vi "deltaHRT.vi"(9 "data input":T3, 10 "Coagulant":T1={"flocculator volume (L)"=100.0, "clarifier volume (L)"=0.0, "dose updates per HRT"=0, "target clarified turbidity (NTU)"=0.3, "Coagulant mode"=enum."manual", "Coag dose [mg/L]"=0.0, "pump mL/rev"=0.0, "clarifier flow [L/s]"=0.5, "min Coag dose [mg/L]"=0.0, "max Coag dose [mg/L]"=0.0, "Steps"=3, "HRT response delay"=1, "Ku*"=1.0} {"HRT response delay" min=1 max=10 step=1; "Steps" min=3 step=1; "clarifier flow [L/s]" min=0.0001 max=1.0 step=0.0001; "target clarified turbidity (NTU)" min=0.1 max=5.0 step=0.01; "dose updates per HRT" min=1 max=100 step=1}, 11 "seconds since 1Jan1904":timestamp) -> (1 "new interval":bool, 2 "sum HRT since dose change":dbl, 3 "total HRT since startup":dbl)   [LabVIEW 2015]
uses:
  coag.ctl
  coag model data.ctl
  model type.ctl
panel:
  out "delta HRT":dbl
  # "min"
  # "max"
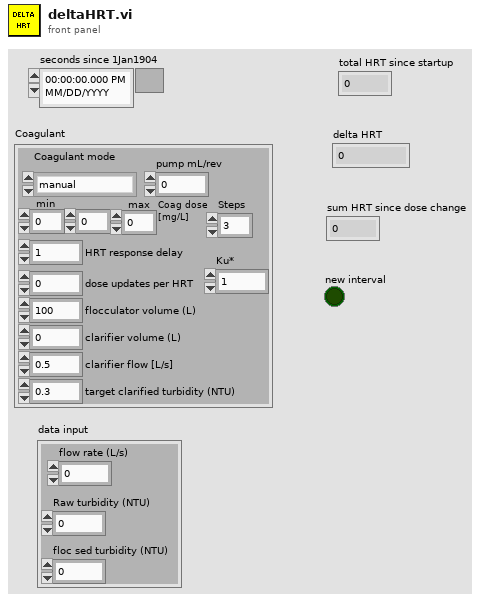
[diagram p1: front panel]
types:
  T1 = typedef "coag.ctl" = cluster{"flocculator volume (L)":dbl, "clarifier volume (L)":dbl, "dose updates per HRT":u16, "target clarified turbidity (NTU)":dbl, "Coagulant mode":T2, "Coag dose [mg/L]":dbl, "pump mL/rev":dbl, "clarifier flow [L/s]":dbl, "min Coag dose [mg/L]":dbl, "max Coag dose [mg/L]":dbl, "Steps":u16, "HRT response delay":u32, "Ku*":dbl}
  T2 = typedef "model type.ctl" = enum16{"manual", "ramp", "simple corrector", "linear regression"}
  T3 = typedef "coag model data.ctl" = cluster{"flow rate (L/s)":dbl, "Raw turbidity (NTU)":dbl, "floc sed turbidity (NTU)":dbl}
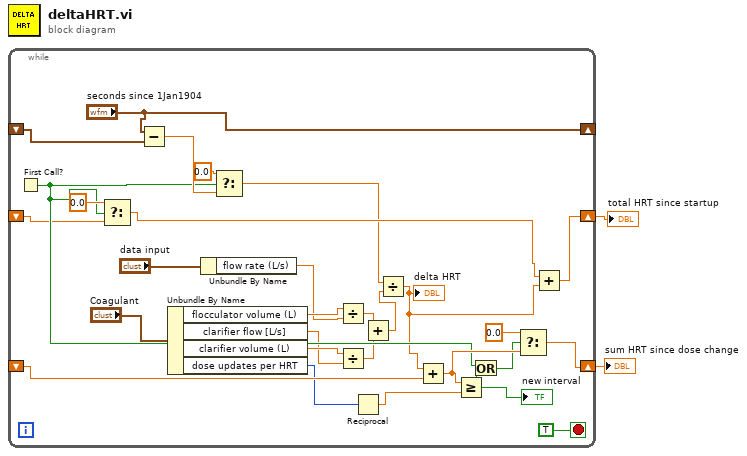
[diagram p0: block diagram]
diagram:
  n1 = while {
    shift-right: ["seconds since 1Jan1904"] -> _
    shift-left: _ -> [w28]
    shift-right: [w23] -> w2
    shift-left: _ -> [w24]
    shift-right: [w18] -> w1
    shift-left: _ -> [w15]
    stop <- TRUE stop-if-true
    n2 = First Call?() -> (First Call?: T/F=w16:bool)
    n3 = Select(t=0.0, s=w16, f=w15) -> (s? t:f=w14:dbl)
    n4 = Subtract(x="seconds since 1Jan1904", y=w28) -> (x-y=w27:dbl)
    n5 = Unbundle By Name("Coagulant") -> ("flocculator volume (L)"=w12:dbl, "clarifier flow [L/s]"=w9:dbl, "clarifier volume (L)"=w10:dbl, "dose updates per HRT"=w13:u16)
    n6 = Unbundle By Name("data input") -> ("flow rate (L/s)"=w11:dbl)
    n7 = Select(t=0.0, s=w16, f=w27) -> (s? t:f=w5:dbl)
    n8 = Divide(x=w12, y=w11) -> (x/y=w8:dbl)
    n9 = Divide(x=w10, y=w9) -> (x/y=w7:dbl)
    n10 = Reciprocal(x=w13) -> (1/x=w19:dbl)
    n11 = Add(x=w8, y=w7) -> (x+y=w6:dbl)
    n12 = Divide(x=w5, y=w6) -> (x/y=w4:dbl)
    "delta HRT" <- w4
    n13 = Add(x=w4, y=w24) -> (x+y=w21:dbl)
    n14 = Greater Or Equal?(x=w21, y=w19) -> (x >= y?=w22:bool)
    "new interval" <- w22
    n15 = Or(x=w16, y=w22) -> (x .or. y?=w20:bool)
    n16 = Select(t=0.0, s=w20, f=w21) -> (s? t:f=w23:dbl)
    n17 = Add(x=w14, y=w4) -> (x+y=w18:dbl)
  }
  "sum HRT since dose change" <- w2
  "total HRT since startup" <- w1
